vi "EnableAlarm.vi"(7 "Cal_Enable":bool, 11 "AlarmThresholds":T1 {"ErrsAndWarns" scale=0.0..10.0}) -> (3 "AlarmThresholds out":T1 {"ErrsAndWarns" scale=0.0..10.0})   [LabVIEW 2018]
uses:
  Controls/Clusts/AlarmThresh_OneChan.ctl
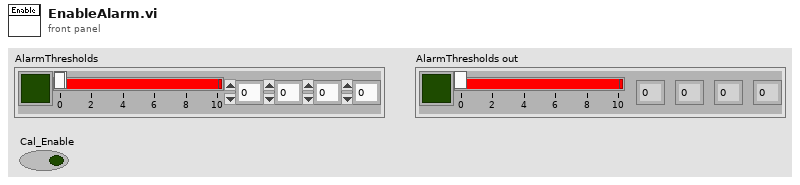
[diagram p1: front panel]
types:
  T1 = typedef "AlarmThresh_OneChan.ctl" = cluster{"Enbl":bool, "ErrsAndWarns":cluster{dbl, dbl, dbl, dbl}}
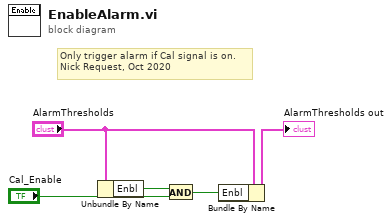
[diagram p0: block diagram]
diagram:
  # "Only trigger alarm if Cal signal is on.\nNick Request, Oct 2020"
  n1 = Unbundle By Name("AlarmThresholds") -> ("Enbl"=w2:bool)
  n2 = And(x=w2, y="Cal_Enable") -> (x .and. y?=w1:bool)
  n3 = Bundle By Name(cluster="AlarmThresholds", "Enbl"=w1) -> (→"AlarmThresholds out":T1)
